vi "Finish.vi"   [LabVIEW 2019]
doc: "This VI is called during exit. It can be used to close I/O refnums, save collected data, etc."
uses:
  <vilib>/Rock Robotics/WPI/Utilities/WPI_GetSetVariantRefNum.vi
types:
  T1 = typedef "WPI_JoystickDevRef.ctl" = cluster{"Device":T2}
  T2 = typedef "WPI_JoystickDeviceEnum.ctl" = enum16{"USB 0", "USB 1", "USB 2", "USB 3", "USB 4", "USB 5"}
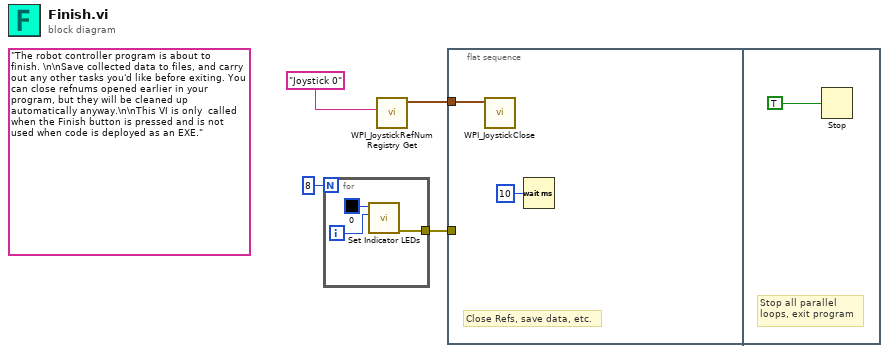
[diagram p0: block diagram]
diagram:
  (unwired) "The robot controller program is about to finish. \n\nSave collected data to files, and carry out any other tasks you'd like before exiting. You can close refnums opened earlier in your program, but they will be cleaned up automatically anyway.\n\nThis VI is only  called when the Finish button is pressed and is not used when code is deployed as an EXE."
  n1 = for {
    N: 8 -> [_]
    tunnel: [w5] -> w1
    i -> [w7]
    n2 = call "Set Indicator LEDs.vi"("LED Index"=w7, "Color"=u32 0) -> ("error out"=w5:errorcluster)  [unwired: 9 in]
  }
  n3 = call <vilib>:"WPI_JoystickRefNum Registry Get.vi"("refnum name"="Joystick 0") -> ("JoystickDevRef"=w3:T1)  [unwired: 1 in, 9 out]
  n4 = flat-sequence {
    tunnel: w3 -> [w9]
    tunnel: w1 -> [_]
    frame #0 {
      # "Close Refs, save data, etc."
      n5 = call <vilib>:"WPI_JoystickClose.vi"("JoystickDevRef"=w9) -> ()  [unwired: 11 out]
      n6 = Wait (ms)(milliseconds to wait=u32 10) -> ()  [unwired: 1 out]
    }
    frame #1 {
      # "Stop all parallel\nloops, exit program"
      n7 = Stop(stop? (T)=TRUE ("Quit")) -> ()
    }
  }
